vi "four_transactions.vi"() -> ()   [LabVIEW 2019]
panel:
  out "çarp":bool
  out "böl":bool
  out "fark":bool
  out "toplam":bool
  in  "Slide":dbl(slide) scale=0.0..3.0
  in  "Sayı1":dbl
  in  "Sayı2":dbl
  in  "stop":bool
  out "sonuc":dbl
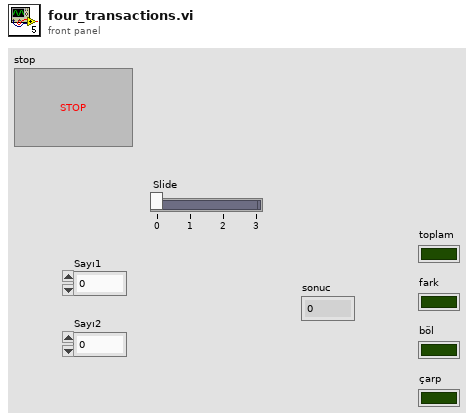
[diagram p1: front panel]
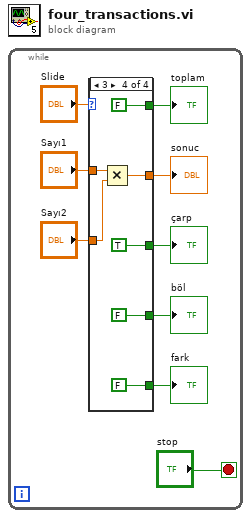
[diagram p0: block diagram]
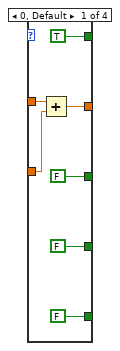
[diagram p2: hidden frame]
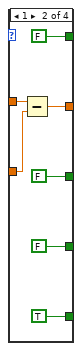
[diagram p3: hidden frame]
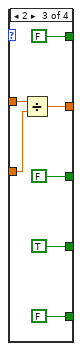
[diagram p4: hidden frame]
diagram:
  n1 = while {
    stop <- "stop" stop-if-true
    n2 = case shown="3" "Slide" {
      tunnel: [w14 w21 w30 w35] -> w8
      tunnel: "Sayı1" -> [w16 w23 w29 w37]
      tunnel: "Sayı2" -> [w15 w22 w28 w36]
      tunnel: [TRUE FALSE FALSE FALSE] -> w4
      tunnel: [FALSE TRUE FALSE FALSE] -> w3
      tunnel: [FALSE FALSE FALSE TRUE] -> w2
      tunnel: [FALSE FALSE TRUE FALSE] -> w1
      frame 0, Default {
        n3 = Add(x=w16, y=w15) -> (x+y=w14:dbl)
      }
      frame 1 {
        n4 = Subtract(x=w23, y=w22) -> (x-y=w21:dbl)
      }
      frame 2 {
        n5 = Divide(x=w29, y=w28) -> (x/y=w30:dbl)
      }
      frame 3 {
        n6 = Multiply(x=w37, y=w36) -> (x*y=w35:dbl)
      }
    }
    "sonuc" <- w8
    "toplam" <- w4
    "fark" <- w3
    "çarp" <- w2
    "böl" <- w1
  }
